vi "FTW-Actor-GetNextJob.vi"(8 "error in":errorcluster, 10 "Jobs Performed":i32, 11 "FTW Actor in":refnum<class "FTW-Actor.lvclass">) -> (0 "error out":errorcluster, 1 "Job Data":string, 2 "Job Name":string, 3 "FTW Actor":refnum<class "FTW-Actor.lvclass">)   [LabVIEW 2013, in "FTW-Actor.lvclass"]
uses:
  FTW-Actor.lvclass
  FTW-Actor.lvclass/FTW-Actor.ctl
  Sequencer/FTW-Sequencer.lvclass/FTW-Sequencer.ctl
  Regex/FTW-Regex.vi
  Error/FTW-ERR-StatusException.vi
  Error/FTW-ERR-Clear.vi
  Error/FTW-ERR-ThrowError.vi
  Sequencer/FTW-Sequencer.lvclass
panel:
  # "Inputs"
  # "Outputs"
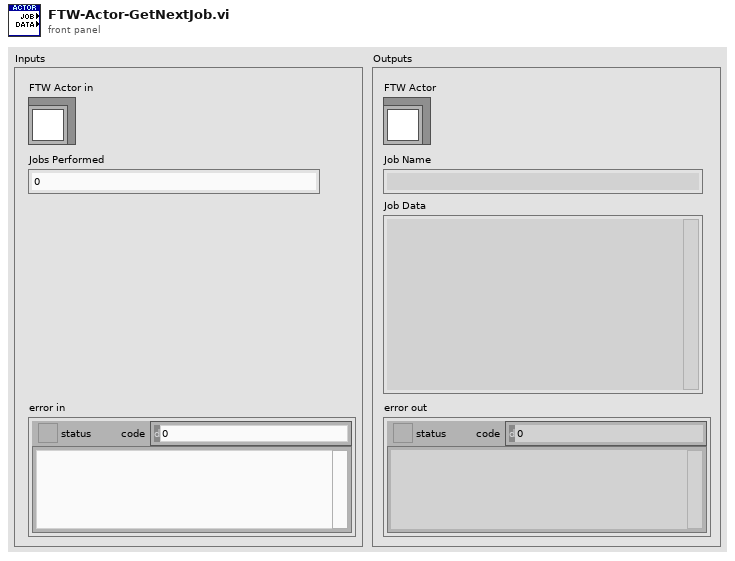
[diagram p1: front panel]
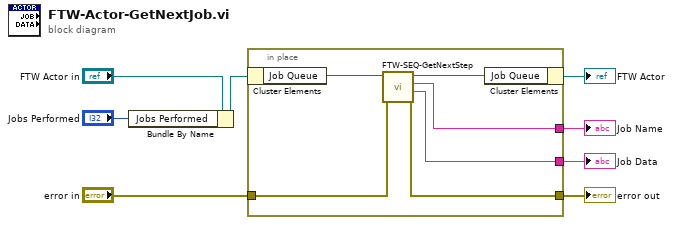
[diagram p0: block diagram]
diagram:
  n1 = Bundle By Name(cluster="FTW Actor in", "Jobs Performed"="Jobs Performed") -> (w2:refnum<class "FTW-Actor.lvclass">)
  n2 = in-place {
    in-place-border: "error in" -> [w14]
    in-place-border: [w13] -> w7
    in-place-border: [w10] -> w4
    in-place-border: [w9] -> w3
    n3 = in-place-cluster #1(w2) -> ("Job Queue"=w12:refnum<class "FTW-Sequencer.lvclass">)
    n4 = call "FTW-SEQ-GetNextStep.vi"("error in"=w14, "Sequencer"=w12) -> ("error out"=w13:errorcluster, "Job Data"=w9:string, "Current Job"=w10:string, "Sequencer out"=w11:refnum<class "FTW-Sequencer.lvclass">)  [unwired: 6 in]
    n5 = in-place-cluster #1("Job Queue"=w11) -> (→"FTW Actor":refnum<class "FTW-Actor.lvclass">)
  }
  "error out" <- w7
  "Job Name" <- w4
  "Job Data" <- w3
